vi "plot_update_cursorPos.vi"(0 "cursor list":T1(array[cluster]) {"Location"."Y" format="%.2f"; "Location"."X" format="%.2f"}, 1 "x zoom factor":dbl format="%.2f", 3 "x min":sgl format="%.2f", 4 "x max":sgl format="%.2f", 5 "error in (no error)":errorcluster, 6 "y max":sgl format="%.2f", 8 "y min":sgl format="%.2f") -> (14 "cursor list out":T1(array[cluster]) {"Location"."Y" format="%.2f"; "Location"."X" format="%.2f"}, 19 "error out":errorcluster)   [LabVIEW 2010, in "OSA.lvclass"]
doc: "SubVI to a <B>Thorlabs_OSA_64</B> object.\n\n[GOOP 1.0]"
uses:
  OSA.lvclass
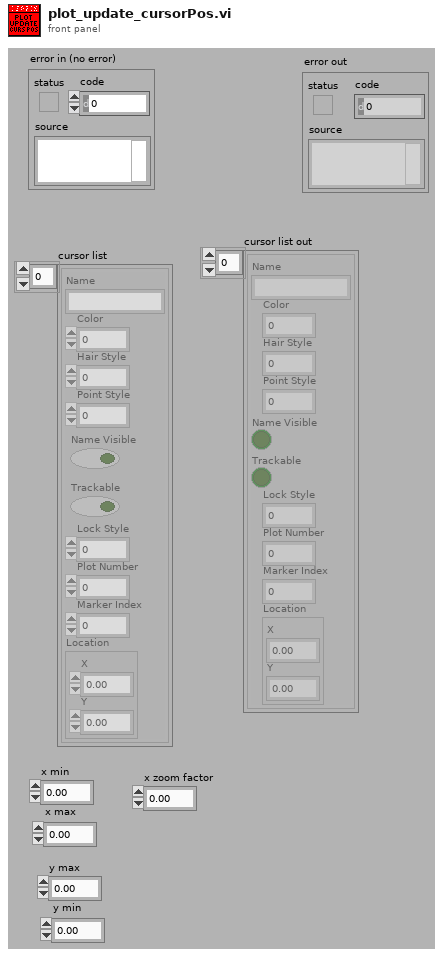
[diagram p1: front panel]
types:
  T1 = cluster{"Name":string, "Color":u32, "Hair Style":u8, "Point Style":u8, "Name Visible":bool, "Trackable":bool, "Lock Style":u32, "Plot Number":u32, "Marker Index":i32, "Location":cluster{"X":dbl, "Y":dbl}}[]
  T2 = cluster{"Name":string, "Color":u32, "Hair Style":u8, "Point Style":u8, "Name Visible":bool, "Trackable":bool, "Lock Style":u32, "Plot Number":u32, "Marker Index":i32, "Location":cluster{"X":dbl, "Y":dbl}}
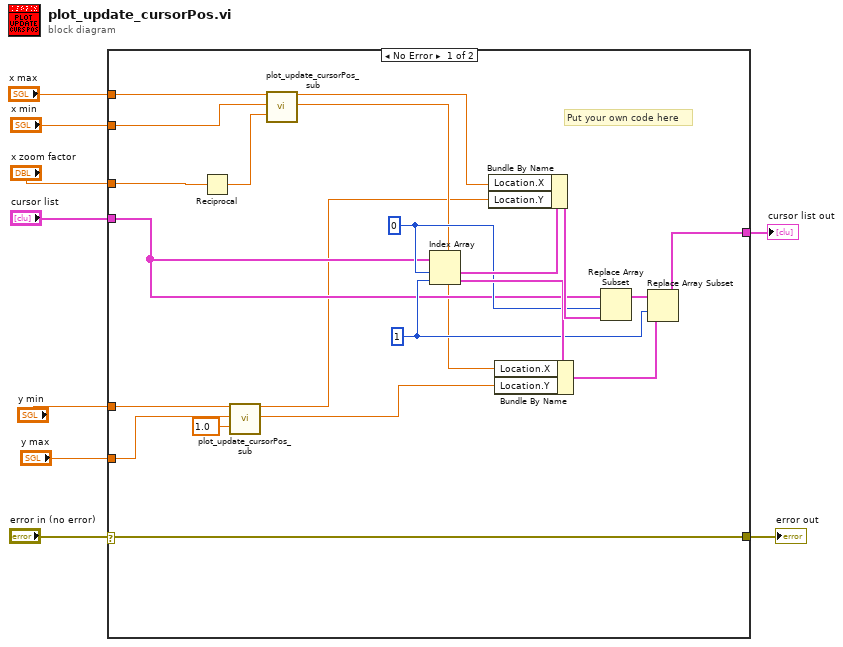
[diagram p0: block diagram]
diagram:
  n1 = case shown="No Error" "error in (no error)" {
    selector: "error in (no error)" -> [w30 w32]
    tunnel: [w30 w32] -> w9
    tunnel: "cursor list" -> [w22 w31]
    tunnel: [w21 w31] -> w6
    tunnel: "x min" -> [w18 _]
    tunnel: "x max" -> [w17 _]
    tunnel: "y min" -> [w16 _]
    tunnel: "y max" -> [w15 _]
    tunnel: "x zoom factor" -> [w10 _]
    frame No Error {
      w23 = 1 ("index")
      w24 = 0 ("index")
      # "Put your own code here"
      n2 = Reciprocal(x=w10) -> (1/x=w11:dbl)
      n3 = call "plot_update_cursorPos_sub.vi"("min"=w16, "max"=w15, "factor"=sgl 1.0) -> ("min"=w13:sgl, "max"=w12:sgl)  [unwired: 15 in]
      n4 = call "plot_update_cursorPos_sub.vi"("min"=w17, "max"=w18, "factor"=w11) -> ("min"=w20:sgl, "max"=w19:sgl)  [unwired: 15 in]
      n5 = Index Array(array=w22, index #1=w24, index #2=w23) -> (element #1=w28:T2, element #2=w27:T2)
      n6 = Bundle By Name(cluster=w28, "Location.X"=w20, "Location.Y"=w13) -> (w29:T2)
      n7 = Bundle By Name(cluster=w27, "Location.X"=w19, "Location.Y"=w12) -> (w25:T2)
      n8 = Replace Array Subset(array=w22, new element=w29, index=w24) -> (w26:T1)
      n9 = Replace Array Subset(array=w26, new element=w25, index=w23) -> (w21:T1)
    }
    frame Error {
      # "Error"
    }
  }
  "error out" <- w9
  "cursor list out" <- w6
